vi "AR Drone - Simple Video.vi"() -> ()   [LabVIEW 2014]
doc: "Very simple example showing how to use the base VIs to control the AR Drone and receive and display video data."
uses:
  <vilib>/LVH/AR Drone Toolkit/AR Drone.lvlib
panel:
  out "Video Stream":picture
  in  "Control Cluster":T1 {"Yaw Speed" scale=-1.0..1.0; "Vertical Speed" scale=-1.0..1.0; "Pitch" scale=-1.0..1.0; "Roll" scale=-1.0..1.0}
  in  "stop":bool
  in  "Emergency Landing":bool
  in  "Take Off/Land":bool
  in  "Hover":bool
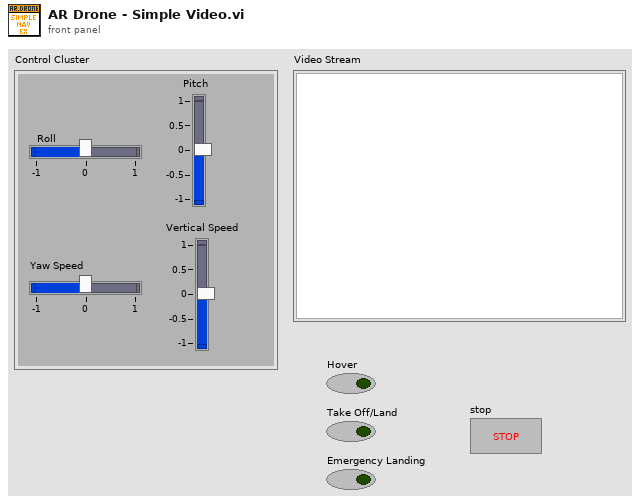
[diagram p1: front panel]
types:
  T1 = cluster{"Roll":sgl, "Pitch":sgl, "Vertical Speed":sgl, "Yaw Speed":sgl}
  T2 = typedef "AR Drone.lvlib/AR Drone Resource.ctl" = cluster{"UDP Control Connection":refnum<k16>, "UDP NavData Connection":refnum<k16>, "UDP Video Connection (Drone 1.0)":refnum<k16>, "TCP Video Connection (Drone 2.0)":refnum<k5>, "TCP Control Port Connection":refnum<k5>, "Drone IP address":string, "Drone Command Port":u16, "Drone NavData Port":u16, "Drone Vid Stream Port":u16, "Drone TCP Control Port":u16, "Home IP address":string, "Home Command Port":u16, "Home NavData Port":u16, "Home Vid Stream Port":u16, "Drone Version":i32}
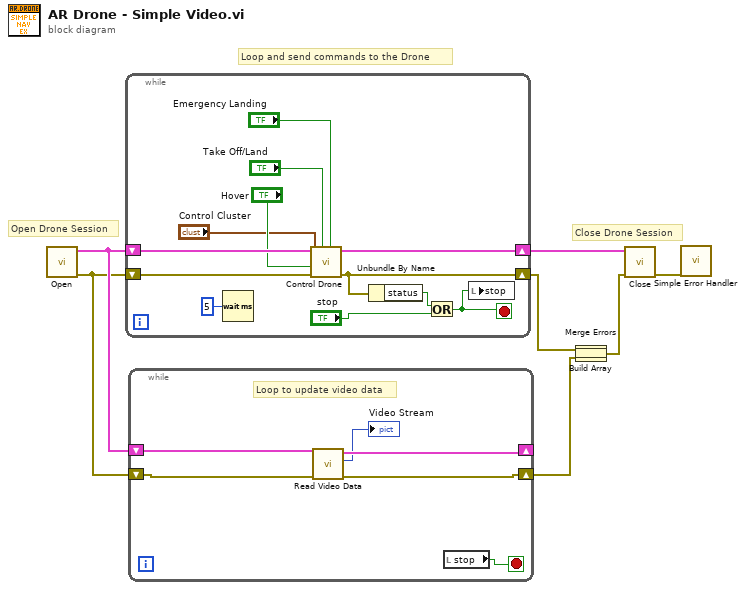
[diagram p0: block diagram]
diagram:
  # "Close Drone Session"
  # "Loop and send commands to the Drone"
  # "Open Drone Session"
  n1 = call <vilib>:"Open.vi"() -> ("error out"=w6:errorcluster, "AR Drone Resource"=w7:T2)  [unwired: 10 in]
  n2 = while {
    shift-right: [w15] -> w8
    shift-left: w7 -> [w19]
    shift-right: [w10] -> w4
    shift-left: w6 -> [w20]
    stop <- w9 stop-if-true
    n3 = Wait (ms)(milliseconds to wait=u32 5) -> ()  [unwired: 1 out]
    n4 = call <vilib>:"Control Drone.vi"("Emergency Landing"="Emergency Landing", "Takeoff/Land"="Take Off/Land", "error in (no error)"=w20, "Hover"="Hover", "Control Cluster"="Control Cluster", "AR Drone Resource"=w19) -> ("error out"=w10:errorcluster, "AR Drone Resource Out"=w15:T2)  [unwired: 4 in]
    n5 = Unbundle By Name(w10) -> ("status"=w12:bool)
    n6 = Or(x=w12, y="stop") -> (x .or. y?=w9:bool)
    n7 = local write "stop"(w9) -> ()
  }
  n8 = while {
    shift-right: [w23] -> _
    shift-left: w7 -> [w25]
    shift-right: [w22] -> w5
    shift-left: w6 -> [w24]
    stop <- w26 stop-if-true
    # "Loop to update video data"
    n9 = call <vilib>:"Read Video Data.vi"("error in (no error)"=w24, "AR Drone Resource"=w25) -> ("error out"=w22:errorcluster, "Video Stream"=→"Video Stream":picture, "AR Drone Resource Out"=w23:T2)  [unwired: 7 in]
    n10 = local read "stop"() -> (w26:bool)
  }
  n11 = Build Array(w4, w5) -> (w1:errorcluster[])
  n12 = Merge Errors(w1) -> (w3:errorcluster)
  n13 = call <vilib>:"Close.vi"("error in (no error)"=w3, "AR Drone Resource"=w8) -> ("error out"=w2:errorcluster)  [unwired: 9 in]
  n14 = call <vilib>:"Simple Error Handler.vi"("error in (no error)"=w2) -> ()  [unwired: 4 in, 5 out]
